vi "IFD Image Position.vi"(5 "Public Denominator":u32, 7 "Basic Unit":T1(ring)=enum."cm", 8 "error in (no error)":errorcluster, 9 "Position":cluster{"X":u32, "Y":u32}, 10 "Pixel Size":cluster{"X":u32, "Y":u32}, 11 "IFD in":refnum<class "IFD.lvclass">) -> (0 "error out":errorcluster, 3 "IFD out":refnum<class "IFD.lvclass">)   [LabVIEW 2016, in "IFD.lvclass"]
uses:
  IFD.lvclass
  Tag/IFD_Tag.lvclass/IFD_Tag.ctl
  IFD.lvclass/IFD.ctl
  Tag/IFD_Tag.lvclass
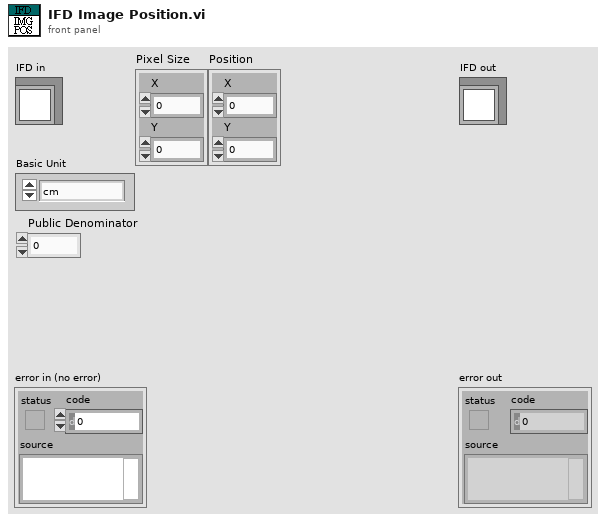
[diagram p1: front panel]
types:
  T1 = enum16{"Undefined(DO NOT USE)", "pixel", "inch", "cm"}
  T2 = enum16{"Undefined(DO NOT USE)", "U8", "ASCII", "U16", "U32", "RATIONAL", "I8", "Undefined 8 bit", "I16", "I32", "SRATIONAL", "SGL", "DBL"}
  T3 = enum16{"big-endian, network order", "native, host order", "little-endian"}
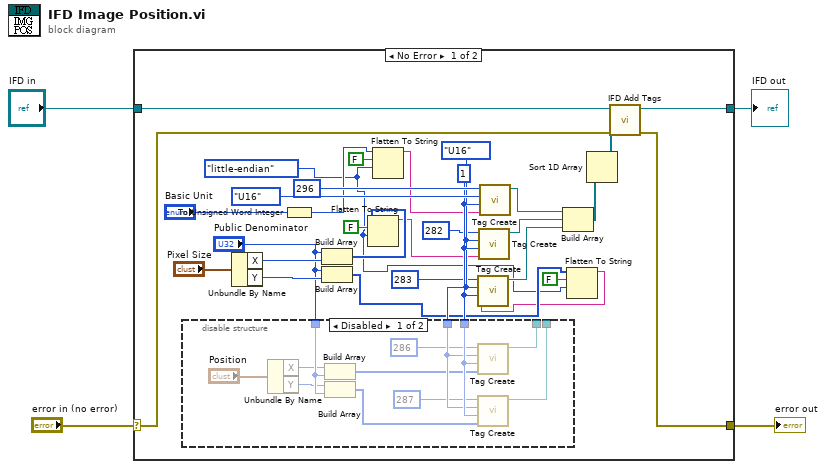
[diagram p0: block diagram]
diagram:
  n1 = case shown="No Error" "error in (no error)" {
    selector: "error in (no error)" -> [w25 w48]
    tunnel: [w24 w48] -> w3
    tunnel: [w33 w47] -> w1
    tunnel: "IFD in" -> [w34 w47]
    frame No Error {
      w5 = T3."little-endian" ("byte order (0:big-endian, network order)")
      w23 = T2."U16" ("Data Type")
      w30 = u32 1 ("Data Count")
      n2 = disable-structure shown="Disabled" {
        disable-tunnel: w30 -> [w46 _]
        disable-tunnel: [w45 _] -> _
        disable-tunnel: [w44 _] -> _
        disable-tunnel: w23 -> [w43 _]
        disable-tunnel: "Public Denominator" -> [w39 _]
        frame Disabled {
          n3 = Unbundle By Name("Position") -> ("X"=w38:u32, "Y"=w37:u32)
          n4 = Build Array(w38, w39) -> (w36:u32[])
          n5 = Build Array(w37, w39) -> (w35:u32[])
          n6 = call "Tag Create.vi"("Data"=w36, "Data Count"=w46, "Data Type"=w43, "Tag ID"=u16 286) -> ("IFD_Tag out"=w45:refnum<class "IFD_Tag.lvclass">)  [unwired: 7 in]
          n7 = call "Tag Create.vi"("Data"=w35, "Data Count"=w46, "Data Type"=w43, "Tag ID"=u16 287) -> ("IFD_Tag out"=w44:refnum<class "IFD_Tag.lvclass">)  [unwired: 7 in]
        }
        frame Enabled {
        }
      }
      n8 = Unbundle By Name("Pixel Size") -> ("X"=w18:u32, "Y"=w17:u32)
      n9 = To Unsigned Word Integer(number="Basic Unit") -> (unsigned 16bit integer=w13:u16)
      n10 = Build Array("Public Denominator", w18) -> (w10:u32[])
      n11 = Build Array("Public Denominator", w17) -> (w7:u32[])
      n12 = Flatten To String(anything=w10, prepend array or string size? (T)=FALSE, byte order (0:big-endian, network order)=w5) -> (data string=w9:string)  [unwired: 1 in, 2 out]
      n13 = Flatten To String(anything=w13, prepend array or string size? (T)=FALSE, byte order (0:big-endian, network order)=w5) -> (data string=w12:string)  [unwired: 1 in, 2 out]
      n14 = call "Tag Create.vi"("Data"=w9, "Data Count"=w30, "Data Type"=w23, "Tag ID"=u16 282) -> ("IFD_Tag out"=w28:refnum<class "IFD_Tag.lvclass">)  [unwired: 7 in]
      n15 = call "Tag Create.vi"("Data"=w12, "Data Count"=w30, "Data Type"=T2."U16", "Tag ID"=u16 296) -> ("IFD_Tag out"=w29:refnum<class "IFD_Tag.lvclass">)  [unwired: 7 in]
      n16 = Flatten To String(anything=w7, prepend array or string size? (T)=FALSE, byte order (0:big-endian, network order)=w5) -> (data string=w6:string)  [unwired: 1 in, 2 out]
      n17 = call "Tag Create.vi"("Data"=w6, "Data Count"=w30, "Data Type"=w23, "Tag ID"=u16 283) -> ("IFD_Tag out"=w27:refnum<class "IFD_Tag.lvclass">)  [unwired: 7 in]
      n18 = Build Array(w29, w28, w27) -> (w26:refnum<class "IFD_Tag.lvclass">[])
      n19 = Sort 1D Array(array=w26) -> (sorted array=w15:refnum<class "IFD_Tag.lvclass">[])
      n20 = call "IFD Add Tags.vi"("error in (no error)"=w25, "Tag(s)"=w15, "IFD in"=w34) -> ("error out"=w24:errorcluster, "IFD out"=w33:refnum<class "IFD.lvclass">)  [unwired: 7 in]
    }
    frame Error {
    }
  }
  "error out" <- w3
  "IFD out" <- w1
